vi "Load Material Theme.vi"(11 "file path":path) -> (0 "error out":errorcluster, 1 "text":string, 2 "Theme":refnum<class "Material Theme.lvclass">)   [LabVIEW 2021, in "TSC Material Theme.lvlib" / "Material Theme.lvclass"]
doc: "Load a material theme from disk in a JSON file format.\n\n<b>Note</b>: legacy XML files from version v4 or below can still be loaded with this VI but should not be saved going forward.\n\n<b>Code Developed By:</b> +\nDaniel Coons +\nTechnology Service Corporation +\nwww.tsc.com/atcs"
uses:
  Material Theme.lvclass
  Material Theme.lvclass/Material Theme.ctl
  8d0b8e92-f2d2-4725-af73-822fbd61956a.vi
  3cd4fc15-787d-41cf-acd3-45f4c7af28a3.vi
  30a1bc54-b62a-49a8-8efc-2c13e9e1dba8.vi
  <vilib>/JDP Science/JSONtext/Next JSON Value.vi
  <vilib>/JDP Science/JSONtext/String Subset.vi
  <vilib>/JDP Science/JSONtext/Parsing/Advance past next JSON Value (inlined COPY).vi
  <vilib>/JDP Science/JSONtext/Parsing/Advance past whitespace.vi
  <vilib>/JDP Science/JSONtext/Parsing/Advance past String.vi
  <vilib>/JDP Science/JSONtext/Parsing/Advance past Number.vi
  <vilib>/JDP Science/JSONtext/Parsing/Advance past Line Ending.vi
  <vilib>/JDP Science/JSONtext/Parsing/Parse Full Path or Item Name.vi
  <vilib>/JDP Science/JSONtext/Parsing/Advance past Array.vi
  <vilib>/JDP Science/JSONtext/Parsing/Advance past Object.vi
  <vilib>/JDP Science/JSONtext/support/Error Cluster From Code.vi
  <vilib>/JDP Science/JSONtext/Offset/Find Item Locations by Path.vi
  <vilib>/JDP Science/JSONtext/JSON text to Variant.vi
  <vilib>/JDP Science/JSONtext/LVClass Serializer/JSONtext LVClass Serializer.lvclass
  Material-Scheme/Material-Scheme.lvclass
  Material-Palette/Material-Palette.lvclass
  <vilib>/JDP Science/JSONtext/JSONtext.lvlib
  TSC Material Theme/TSC Material Theme.lvlib
panel:
  # "FOR DEBUG"
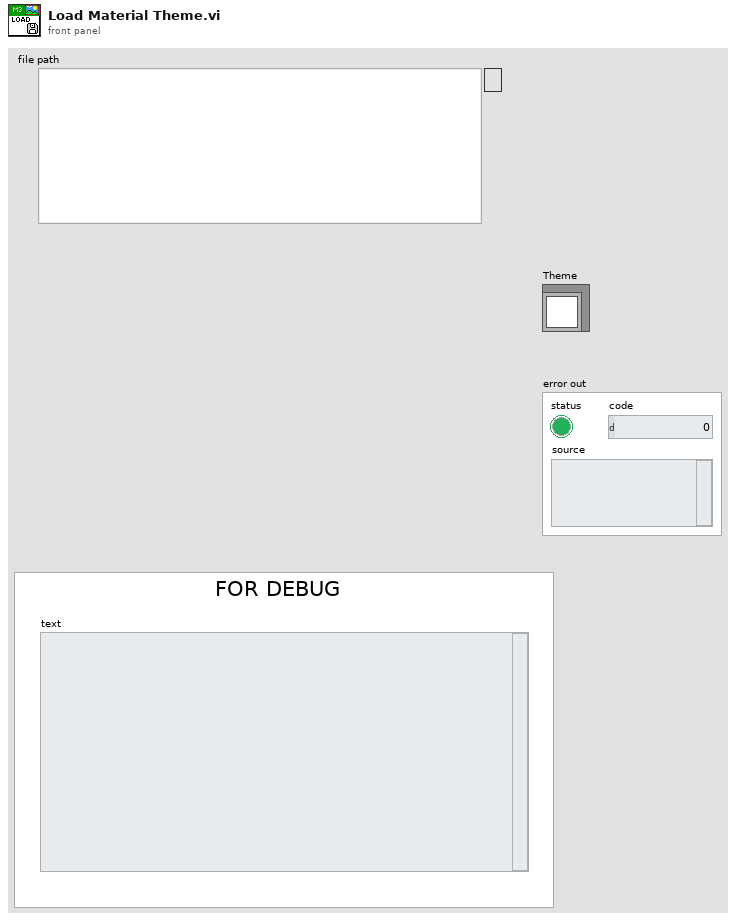
[diagram p1: front panel]
types:
  T1 = cluster{"primary":u32, "secondary":u32, "tertiary":u32, "error":u32}
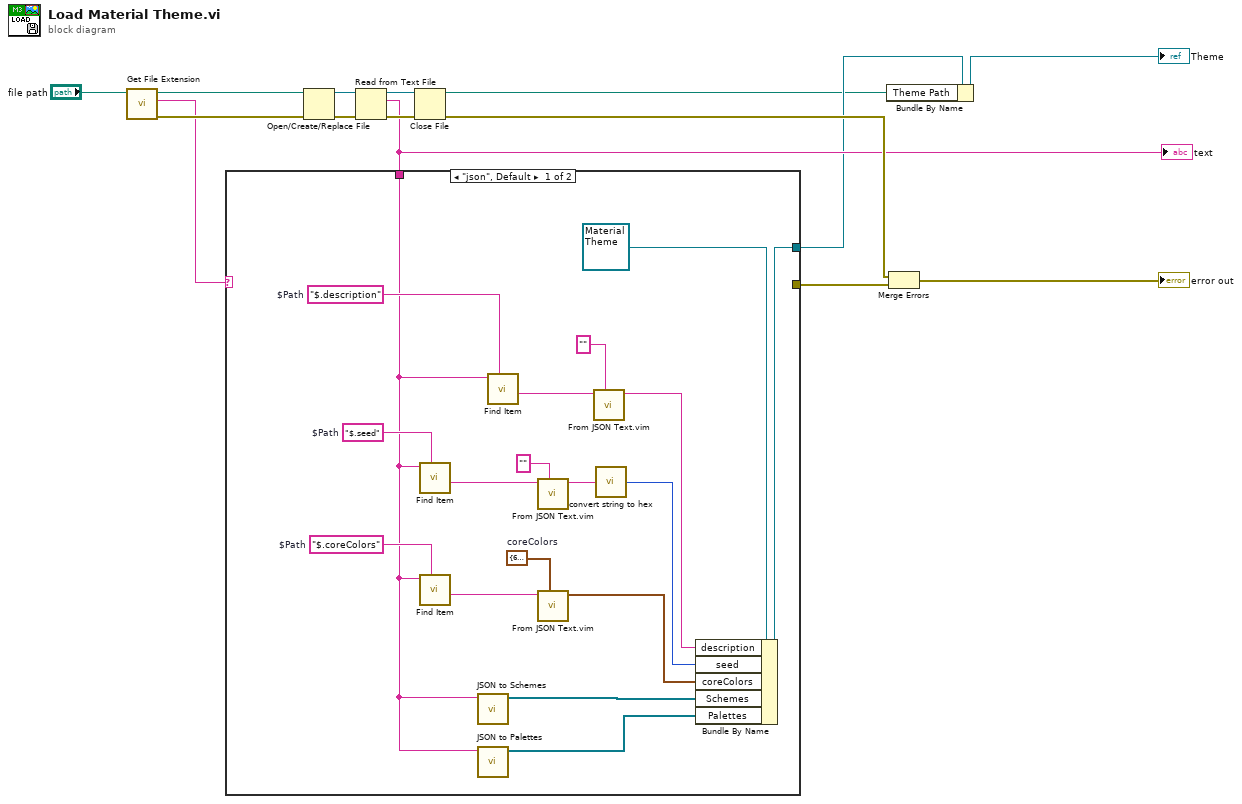
[diagram p0: block diagram]
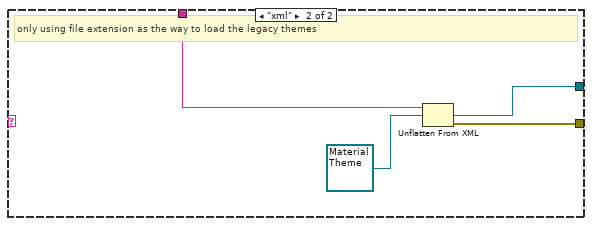
[diagram p2: hidden frame]
diagram:
  n1 = call <vilib>:"Get File Extension.vi"("file"="file path") -> ("error out"=w10:errorcluster, "lowercase file extension"=w1:string, "dup file"=w2:path)  [unwired: 6 in, 2 out]
  n2 = Open/Create/Replace File(file path (use dialog)=w2, error in=w10) -> (refnum out=w9:refnum<file>, error out=w15:errorcluster)  [unwired: 4 in, 1 out]
  n3 = Read from Text File(file (use dialog)=w9, error in=w15) -> (refnum out=w8:refnum<file>, text=w7:string, error out=w14:errorcluster)  [unwired: 2 in, 1 out]
  "text" <- w7
  n4 = case shown="\"json\", Default" w1 {
    tunnel: [_ w37] -> w11
    tunnel: w7 -> [w19 w36]
    tunnel: [w32 w34] -> w5
    frame "json", Default {
      w20 = "$.coreColors"  # $Path
      w17 = T1 {"primary"=6641039, "secondary"=6445937, "tertiary"=8213088, "error"=11740702}  # coreColors
      w27 = "$.seed"  # $Path
      w29 = "$.description"  # $Path
      n5 = call <vilib>:"Find Item.vi"("$Path or Item Name"=w27, "JSON"=w19) -> ("<JSON>"=w25:string)  [unwired: 6 in, 3 out]
      n6 = call <vilib>:"Find Item.vi"("$Path or Item Name"=w20, "JSON"=w19) -> ("<JSON>"=w18:string)  [unwired: 6 in, 3 out]
      n7 = call "JSON to Schemes.vi"("Material JSON"=w19) -> ("Schemes"=w21:refnum<class "Material-Scheme.lvclass">[])  [unwired: 9 in, 1 out]
      n8 = call "JSON to Palettes.vi"("Material JSON"=w19) -> ("Palettes"=w22:refnum<class "Material-Palette.lvclass">[])  [unwired: 9 in, 1 out]
      n9 = call <vilib>:"Find Item.vi"("$Path or Item Name"=w29, "JSON"=w19) -> ("<JSON>"=w31:string)  [unwired: 6 in, 3 out]
      n10 = call "From JSON Text.vim"("Data Type and Default Value"="", "JSON"=w25) -> ("Data out"=w24:string)  [unwired: 8 in, 1 out]
      n11 = call "From JSON Text.vim"("Data Type and Default Value"=w17, "JSON"=w18) -> ("Data out"=w16:T1)  [unwired: 8 in, 1 out]
      n12 = call "From JSON Text.vim"("Data Type and Default Value"="", "JSON"=w31) -> ("Data out"=w28:string)  [unwired: 8 in, 1 out]
      n13 = call "convert string to hex.vi"("string"=w24) -> ("hex"=w23:u32)
      n14 = Bundle By Name(cluster=refnum<class "Material Theme.lvclass"> refnum ("output cluster"), "description"=w28, "seed"=w23, "coreColors"=w16, "Schemes"=w21, "Palettes"=w22) -> (w32:refnum<class "Material Theme.lvclass">)
    }
    frame "xml" {
      # "only using file extension as the way to load the legacy themes"
      n15 = Unflatten From XML(xml string=w36, type=refnum<class "Material Theme.lvclass"> refnum ("output cluster")) -> (value=w34:refnum<class "Material Theme.lvclass">, error out=w37:errorcluster)  [unwired: 1 in]
    }
  }
  n16 = Close File(refnum=w8, error in=w14) -> (path=w3:path, error out=w13:errorcluster)
  n17 = Bundle By Name(cluster=w5, "Theme Path"=w3) -> (→"Theme":refnum<class "Material Theme.lvclass">)
  n18 = Merge Errors(w13, w11) -> (→"error out":errorcluster)
